vi "ICM Config File Path.vi"(8 "error in (no error)":errorcluster) -> (0 "error out":errorcluster, 3 "ICM Config Path":path)   [LabVIEW 2018]
doc: "ICM Config File Path.vi\n\nThis VI defines where the ICM Config Files are stored.\n\nInstrument Communication Module Version 1.0\nJuly, 2017 Original Code Consulting David Thomson\n www.originalcode.com"
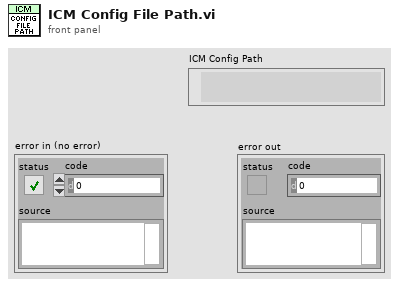
[diagram p1: front panel]
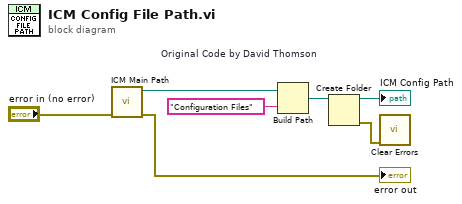
[diagram p0: block diagram]
diagram:
  w7 = "Configuration Files"  # Original Code by David Thomson
  n1 = call "ICM Main Path.vi"("error in (no error)"="error in (no error)") -> ("error out"=→"error out":errorcluster, "ICM Root Path"=w6:path)  [unwired: 8 in, 1 out]
  n2 = Build Path(base path=w6, name or relative path=w7) -> (appended path=w4:path)
  n3 = Create Folder(path (use dialog)=w4) -> (created path=→"ICM Config Path":path, error out=w1:errorcluster)  [unwired: 2 in, 1 out]
  n4 = call "Clear Errors.vi"("error in (no error)"=w1) -> ()  [unwired: 5 in, 2 out]
